vi "Configure Calc Scale.vi"(5 "Scaling Constant B (0)":dbl min=-999999000000.0 max=999999000000.0 step=1e-15 format="%_6g", 6 "Scaling Constant C (1)":dbl=1.0 min=-999999000000.0 max=999999000000.0 step=1e-15 format="%_6g", 7 "Scaling Constant A (1)":dbl=1.0 min=-1000000000000.0 max=1000000000000.0 step=1e-15 format="%_6g", 8 "error in (no error)":errorcluster, 10 "Calculate Scaling  (0: Off)":u16(ring) format="%#.0g" items=["Off", "On"], 11 "VISA resource name":refnum<visa-resource-name>) -> (0 "error out":errorcluster, 3 "VISA resource name out":refnum<visa-resource-name>)   [LabVIEW 2017, in "ADCMT7451_ADC.lvlib"]
doc: "Enables or disables scaling calculation."
uses:
  ADCMT7451_ADC.lvlib
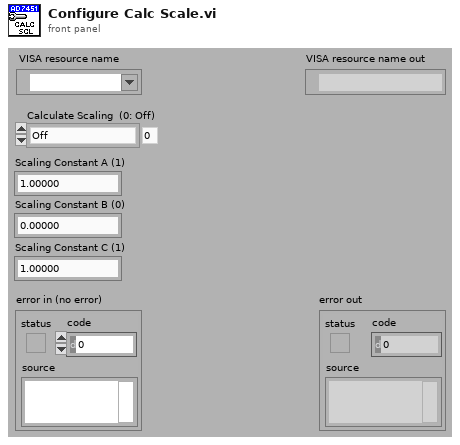
[diagram p1: front panel]
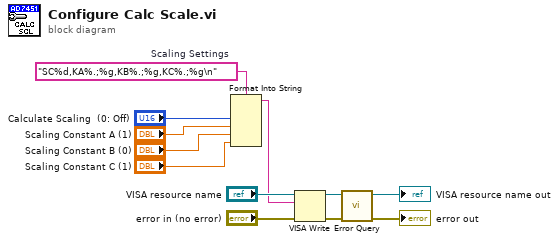
[diagram p0: block diagram]
diagram:
  w6 = "SC%d,KA%.;%g,KB%.;%g,KC%.;%g\n"  # Scaling Settings
  n1 = Format Into String(format string=w6, "Calculate Scaling  (0: Off)", "Scaling Constant A (1)", "Scaling Constant B (0)", "Scaling Constant C (1)") -> (resulting string=w1:string)  [unwired: 2 in, 1 out]
  n2 = VISA Write(VISA resource name="VISA resource name", write buffer=w1, error in (no error)="error in (no error)") -> (VISA resource name out=w8:refnum<visa-resource-name>, error out=w7:errorcluster)  [unwired: 1 out]
  n3 = call "Error Query.vi"("error in (no error)"=w7, "VISA resource name"=w8) -> ("error out"=→"error out":errorcluster, "VISA resource name out"=→"VISA resource name out":refnum<visa-resource-name>)  [unwired: 6 in, 2 out]
